vi "Write Run Mode.vi"(8 "error in (no error)":errorcluster, 10 "Run Mode":T1, 11 "ProjectBase in":refnum<class "Project.lvclass">) -> (0 "error out":errorcluster, 3 "ProjectBase out":refnum<class "Project.lvclass">)   [LabVIEW 2015, in "Project.lvclass"]
uses:
  Project.lvclass
  RUN_MODE_TYPEDEF.ctl
  Project.lvclass/Project.ctl
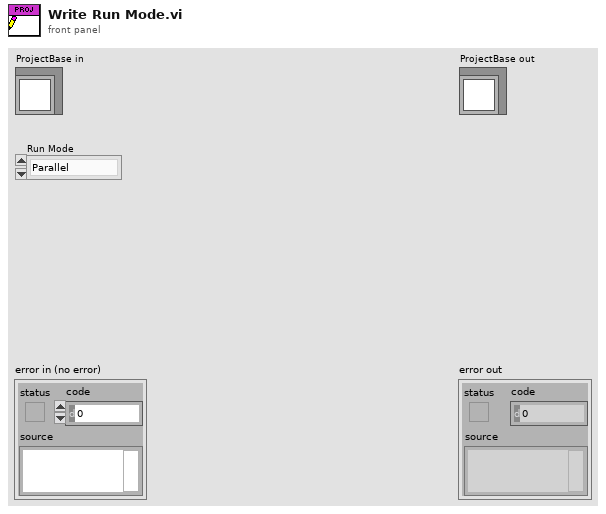
[diagram p1: front panel]
types:
  T1 = typedef "Project.lvclass/RUN_MODE_TYPEDEF.ctl" = enum16{"Parallel", "Batch"}
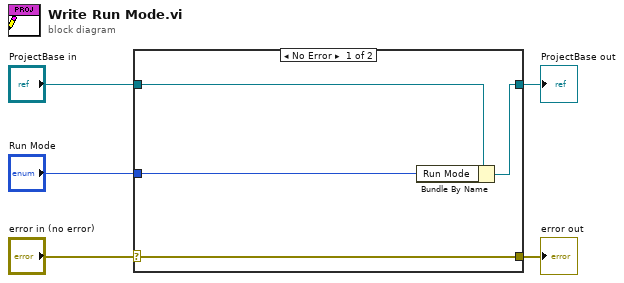
[diagram p0: block diagram]
diagram:
  n1 = case shown="No Error" "error in (no error)" {
    selector: "error in (no error)" -> [w9 w10]
    tunnel: [w9 w10] -> w4
    tunnel: [w7 w11] -> w2
    tunnel: "ProjectBase in" -> [w8 w11]
    tunnel: "Run Mode" -> [w6 _]
    frame No Error {
      n2 = Bundle By Name(cluster=w8, "Run Mode"=w6) -> (w7:refnum<class "Project.lvclass">)
    }
    frame Error {
    }
  }
  "error out" <- w4
  "ProjectBase out" <- w2
